vi "Status Current Stirrer.vi"(8 "error in (no error)":errorcluster, 11 "heater_explorer in":refnum<class "heater_explorer.lvclass">) -> (0 "error out":errorcluster, 2 "Stirrer Option":i32=1 min=1 max=3 step=1, 3 "heater_explorer out":refnum<class "heater_explorer.lvclass">)   [LabVIEW 2020, in "polar_bear_plus_drivers.lvlib" / "heater_explorer.lvclass"]
doc: "Gets the current stirrer selected out of 1 = magnetic (internal, default), 2 = Overhead (small), 3 = Overhead (large) or Tumble Stirrer."
uses:
  <instrlib>/RxnRover/Driver Polar Bear Plus/heater_explorer/heater_explorer.lvclass
  <instrlib>/RxnRover/Driver Polar Bear Plus/heater_explorer/heater_explorer.lvclass/heater_explorer.ctl
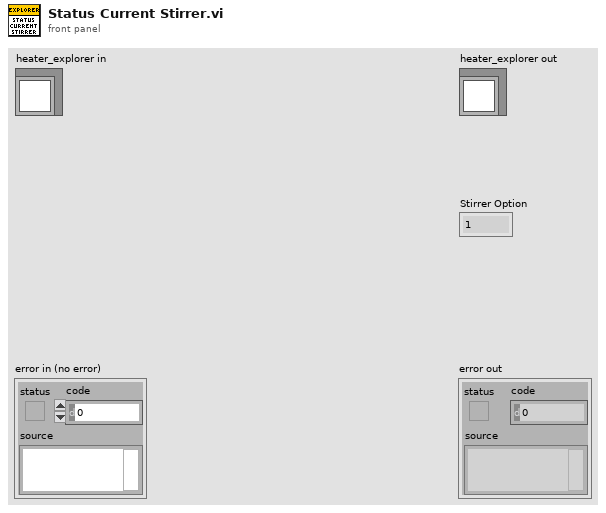
[diagram p1: front panel]
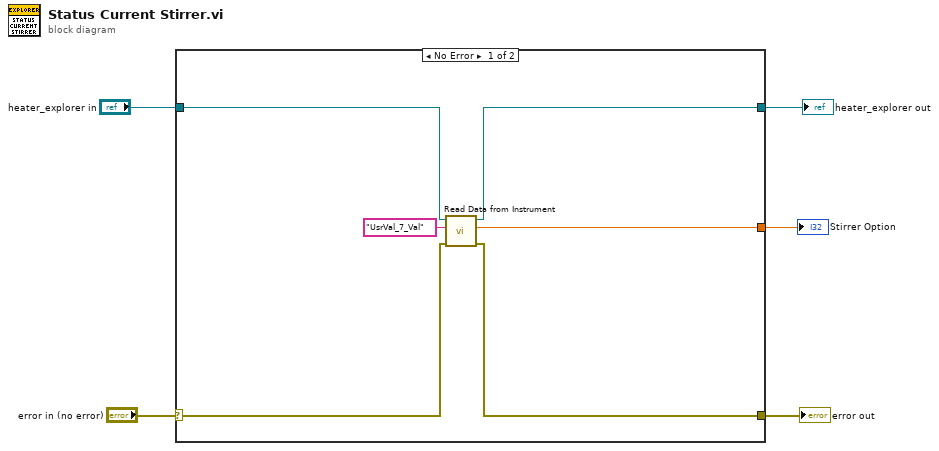
[diagram p0: block diagram]
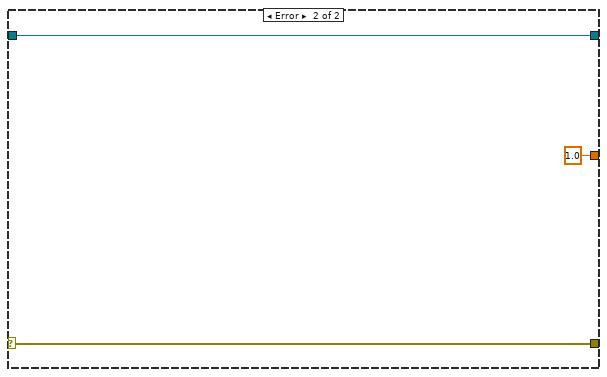
[diagram p2: hidden frame]
diagram:
  n1 = case shown="No Error" "error in (no error)" {
    selector: "error in (no error)" -> [w11 w13]
    tunnel: [w10 w13] -> w4
    tunnel: [w9 1.0 ("Value Read")] -> w3
    tunnel: "heater_explorer in" -> [w7 w14]
    tunnel: [w6 w14] -> w1
    frame No Error {
      n2 = call-dynamic "Read Data from Instrument.vi"("error in (no error)"=w11, "Address"="UsrVal_7_Val", "heater_parent in"=w7) -> ("error out"=w10:errorcluster, "Value Read"=w9:dbl, "heater_parent out"=w6:refnum<class "heater_explorer.lvclass">)  [unwired: 6 in]
    }
    frame Error {
    }
  }
  "error out" <- w4
  "heater_explorer out" <- w1
  "Stirrer Option" <- w3
